vi "REPORT_CBATCH_prepare_header_for_csv.vi"(11 "REPORT_CBATCH_all_info":T1) -> (3 "report_header":string[][](array[string]))   [LabVIEW 2019]
uses:
  typedef/REPORT_CBATCH_all_info.ctl
  DATES/typedef/REPORT_DATES_statuses.ctl
  _misc/AULocalize/SubVIs/Get Localized Phrase Compact Interface 1D.vi
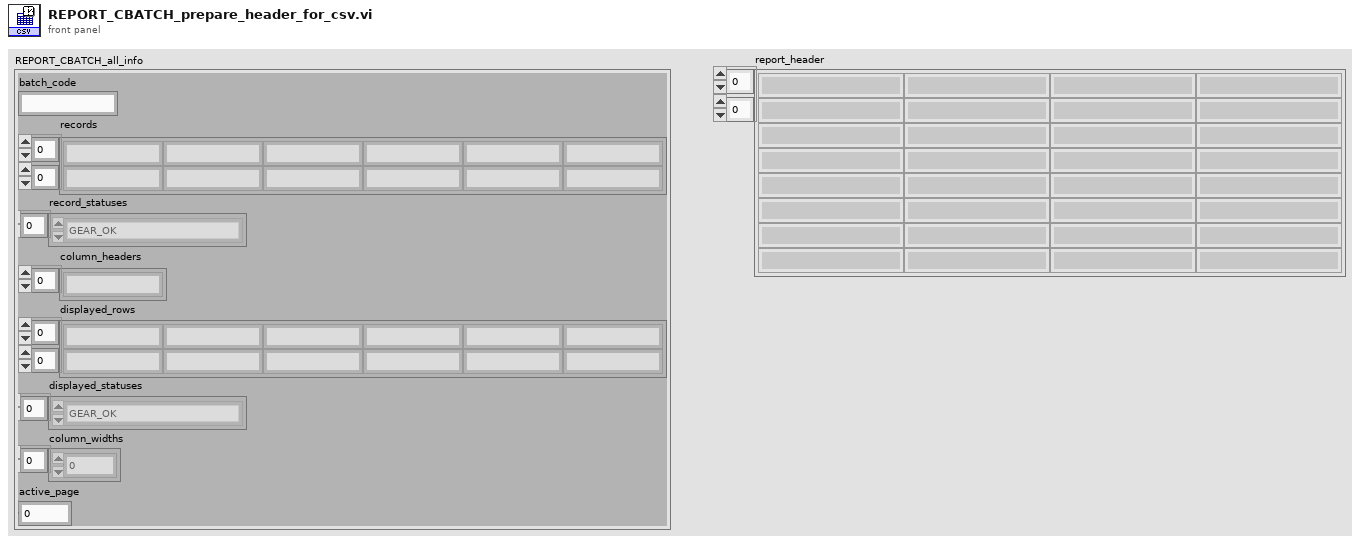
[diagram p1: front panel]
types:
  T1 = typedef "REPORT_CBATCH_all_info.ctl" = cluster{"batch_code":string, "records":string[][], "record_statuses":T2[], "column_headers":string[], "displayed_rows":string[][], "displayed_statuses":T2[], "column_widths":i16[], "active_page":i32}
  T2 = typedef "REPORT_DATES_statuses.ctl" = enum16{"GEAR_OK", "GEAR_NOK", "GEAR_interrupted", "GEAR_in_operation", "GEAR_unexpected"}
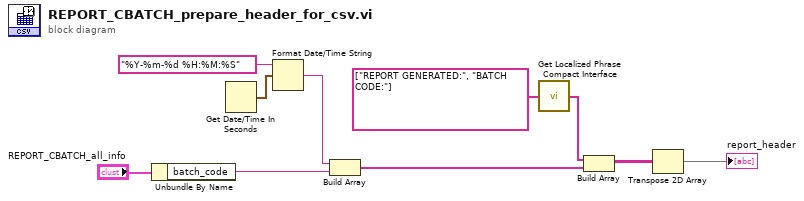
[diagram p0: block diagram]
diagram:
  n1 = Unbundle By Name("REPORT_CBATCH_all_info") -> ("batch_code"=w2:string)
  n2 = Get Date/Time In Seconds() -> (seconds since 1Jan1904=w9:timestamp)
  n3 = Format Date/Time String(time format string (%c)="%Y-%m-%d %H:%M:%S", seconds (now)=w9) -> (date/time string=w3:string)  [unwired: 1 in]
  n4 = Build Array(w3, w2) -> (w4:string[])
  n5 = call-poly "Get Localized Phrase Compact Interface.vi"("Key"=string[] ["REPORT GENERATED:", "BATCH CODE:"]) -> ("Translated Phrase"=w1:string[])
  n6 = Build Array(w1, w4) -> (w7:string[][])
  n7 = Transpose 2D Array(2D array=w7) -> (transposed array=→"report_header":string[][])
